vi "GetSeqPoly.vi"   [LabVIEW 2022 SP3]
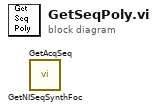
[diagram p0: block diagram]
diagram:
  n1 = call "GetNISeqSynthFoc.vi"() -> ()  [unwired: 21 in, 7 out]
  n2 = call "GetAcqSeq.vi"() -> ()  [unwired: 22 in, 6 out]
